vi "Write cell Data.vi"(8 "error in":errorcluster, 10 "PAS Cell Data in":refnum<class "PAS Cell Data.lvclass">, 11 "PAS File Obs in":refnum<class "PAS File Obs.lvclass">) -> (0 "error out":errorcluster, 3 "PAS File Obs out":refnum<class "PAS File Obs.lvclass">)   [LabVIEW 2015, in "PAS File Obs.lvclass"]
uses:
  PAS File Obs.lvclass
  Data/Cell/PAS Cell Data.lvclass
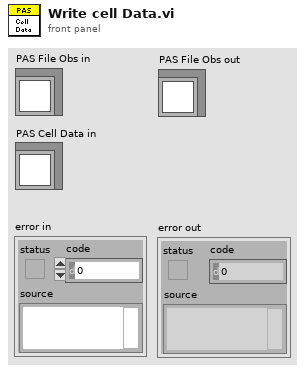
[diagram p1: front panel]
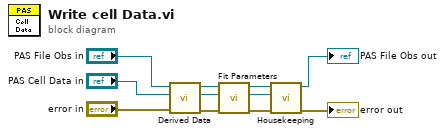
[diagram p0: block diagram]
diagram:
  n1 = call "Derived Data.vi"("error in"="error in", "PAS Cell Data in"="PAS Cell Data in", "PAS File Obs in"="PAS File Obs in") -> ("error out"=w6:errorcluster, "PAS Cell Data Out"=w7:refnum<class "PAS Cell Data.lvclass">, "PAS File Obs Out"=w8:refnum<class "PAS File Obs.lvclass">)  [unwired: 6 in]
  n2 = call "Fit Parameters.vi"("error in"=w6, "PAS Cell Data in"=w7, "PAS File Obs in"=w8) -> ("error out"=w10:errorcluster, "PAS Cell Data Out"=w9:refnum<class "PAS Cell Data.lvclass">, "PAS File Obs Out"=w11:refnum<class "PAS File Obs.lvclass">)  [unwired: 6 in]
  n3 = call "Housekeeping.vi"("error in"=w10, "PAS Cell Data In"=w9, "PAS File Obs in"=w11) -> ("error out"=→"error out":errorcluster, "PAS File Obs Out"=→"PAS File Obs out":refnum<class "PAS File Obs.lvclass">)  [unwired: 6 in, 1 out]
